vi "Average_Corner.vi"(7 "Average\nProjection":bool, 8 "Image":dbl[][](graph), 9 "Cursor C Coordinate":cluster{"X":dbl, "Y":dbl}, 10 "Cursor B Coordinate":cluster{"X":dbl, "Y":dbl}, 11 "Cursor A Coordinate":cluster{"X":dbl, "Y":dbl}) -> (0 "Cut image":dbl[][](graph), 1 "X-Axis":dbl[](array[numeric]), 2 "Intensity Average":dbl[](array[numeric]), 3 "Average\ncut image":dbl)   [LabVIEW 2014]
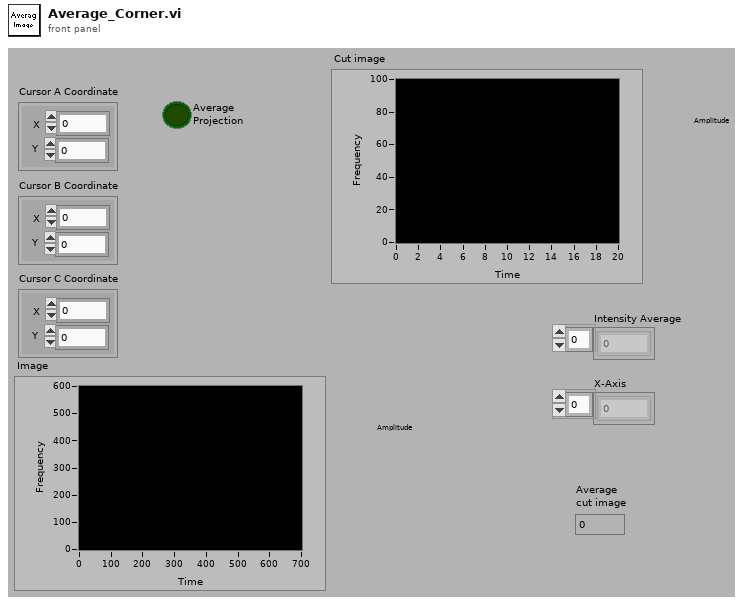
[diagram p1: front panel]
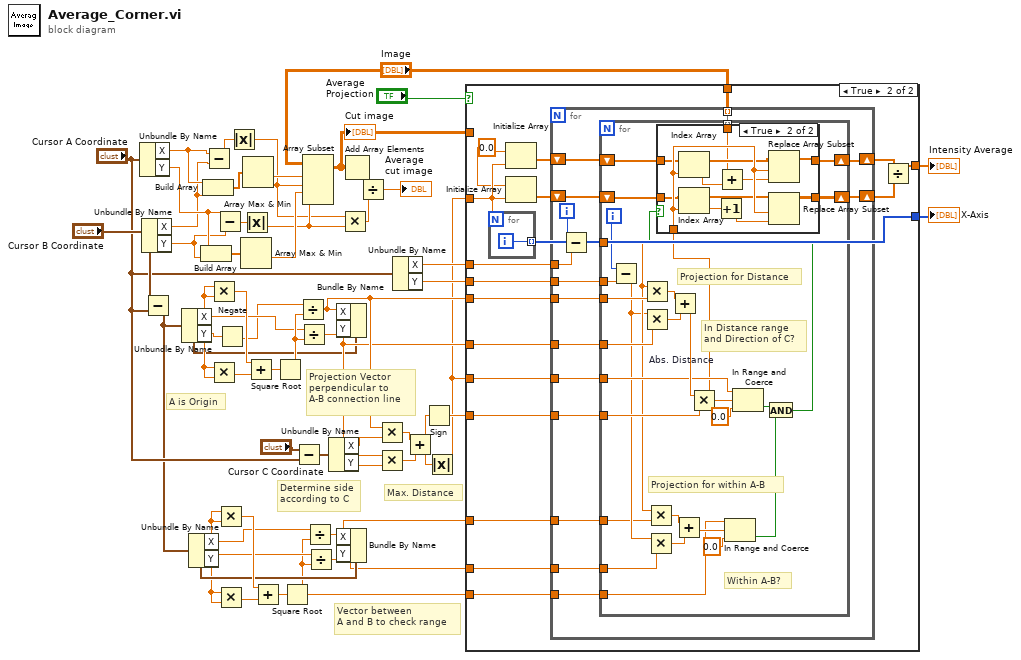
[diagram p0: block diagram]
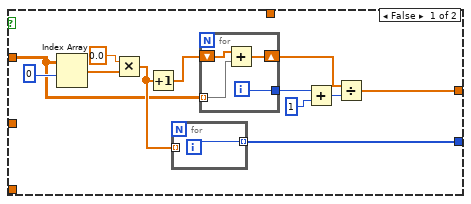
[diagram p2: hidden frame]
diagram:
  # "Vector between\nA and B to check range"
  # "Max. Distance"
  # "Determine side\naccording to C"
  # "A is Origin"
  # "Projection Vector\nperpendicular to \nA-B connection line"
  n1 = Unbundle By Name("Cursor A Coordinate") -> ("X"=w41:dbl, "Y"=w40:dbl)
  n2 = Unbundle By Name("Cursor B Coordinate") -> ("X"=w38:dbl, "Y"=w39:dbl)
  n3 = Subtract(x="Cursor B Coordinate", y="Cursor A Coordinate") -> (x-y=w10:cluster{"X":dbl, "Y":dbl})
  n4 = Unbundle By Name(w10) -> ("X"=w9:dbl, "Y"=w31:dbl)
  n5 = Unbundle By Name(w10) -> ("X"=w6:dbl, "Y"=w7:dbl)
  n6 = Build Array(w40, w39) -> (w50:dbl[])
  n7 = Build Array(w41, w38) -> (w51:dbl[])
  n8 = Subtract(x=w41, y=w38) -> (x-y=w46:dbl)
  n9 = Multiply(x=w9, y=w9) -> (x*y=w29:dbl)
  n10 = Multiply(x=w31, y=w31) -> (x*y=w30:dbl)
  n11 = Subtract(x=w40, y=w39) -> (x-y=w47:dbl)
  n12 = Multiply(x=w6, y=w6) -> (x*y=w11:dbl)
  n13 = Multiply(x=w7, y=w7) -> (x*y=w5:dbl)
  n14 = Negate(x=w31) -> (-x=w8:dbl)
  n15 = Absolute Value(x=w46) -> (abs(x)=w43:dbl)
  n16 = Array Max & Min(array=w50) -> (min value=w48:dbl)  [unwired: 3 out]
  n17 = Absolute Value(x=w47) -> (abs(x)=w44:dbl)
  n18 = Array Max & Min(array=w51) -> (min value=w49:dbl)  [unwired: 3 out]
  n19 = Add(x=w29, y=w30) -> (x+y=w28:dbl)
  n20 = Add(x=w11, y=w5) -> (x+y=w4:dbl)
  n21 = Square Root(x=w28) -> (sqrt(x)=w27:dbl)
  n22 = Square Root(x=w4) -> (sqrt(x)=w1:dbl)
  n23 = Subtract(x="Cursor C Coordinate", y="Cursor A Coordinate") -> (x-y=w20:cluster{"X":dbl, "Y":dbl})
  n24 = Divide(x=w8, y=w27) -> (x/y=w17:dbl)
  n25 = Divide(x=w9, y=w27) -> (x/y=w16:dbl)
  n26 = Array Subset(array="Image", index (row)=w49, length (row)=w43, index (col)=w48, length (col)=w44) -> (w36:dbl[][])
  "Cut image" <- w36
  n27 = Divide(x=w6, y=w1) -> (x/y=w3:dbl)
  n28 = Divide(x=w7, y=w1) -> (x/y=w2:dbl)
  n29 = Unbundle By Name(w20) -> ("X"=w18:dbl, "Y"=w19:dbl)
  n30 = Bundle By Name(cluster=w10, "X"=w17, "Y"=w16) -> ()  [unwired: 1 out]
  n31 = Bundle By Name(cluster=w10, "X"=w3, "Y"=w2) -> ()  [unwired: 1 out]
  n32 = Multiply(x=w43, y=w44) -> (x*y=w42:dbl)
  n33 = Add Array Elements(numeric array=w36) -> (sum=w45:dbl)
  n34 = Divide(x=w45, y=w42) -> (x/y=→"Average\ncut image":dbl)
  n35 = Multiply(x=w17, y=w18) -> (x*y=w22:dbl)
  n36 = Multiply(x=w16, y=w19) -> (x*y=w21:dbl)
  n37 = Unbundle By Name("Cursor A Coordinate") -> ("X"=w24:dbl, "Y"=w23:dbl)
  n38 = Add(x=w22, y=w21) -> (x+y=w14:dbl)
  n39 = Sign(1:w14) -> (0:w15:dbl)
  n40 = Absolute Value(x=w14) -> (abs(x)=w13:dbl)
  n41 = case shown="True" "Average\nProjection" {
    tunnel: w36 -> [w54 _]
    tunnel: [w53 w72] -> w35
    tunnel: [w52 w79] -> w34
    tunnel: w24 -> [_ w86]
    tunnel: w23 -> [_ w85]
    tunnel: w16 -> [_ w84]
    tunnel: w17 -> [_ w83]
    tunnel: w15 -> [_ w82]
    tunnel: w13 -> [_ w81]
    tunnel: w13 -> [_ w80]
    tunnel: "Image" -> [_ w75]
    tunnel: w3 -> [_ w71]
    tunnel: w2 -> [_ w70]
    tunnel: w1 -> [_ w69]
    frame False {
      n42 = Index Array(array=w54, index (row)=u32 0 ("Active Cursor")) -> (element=w56:dbl[])  [unwired: 1 in]
      n43 = Multiply(x=0.0 ("element"), y=w56) -> (x*y=w55:dbl[])
      n44 = Increment(x=w55) -> (x+1=w62:dbl[])
      n45 = for {
        tunnel: w55 -> [_] mode=indexing
        tunnel: [w64] -> w52 mode=indexing
        i -> [w64]
      }
      n46 = for {
        tunnel: w54 -> [w67] mode=indexing
        shift-right: [w66] -> w63
        shift-left: w62 -> [w68]
        tunnel: [w65] -> w59
        i -> [w65]
        n47 = Add(x=w68, y=w67) -> (x+y=w66:dbl[])
      }
      n48 = Add(x=w59, y=u32 1 ("Active Cursor")) -> (x+y=w61:u32)
      n49 = Divide(x=w63, y=w61) -> (x/y=w53:dbl[])
    }
    frame True {
      w76 = 0.0
      n50 = for {
        N: w80 -> [_]
        tunnel: [w87] -> w79 mode=indexing
        i -> [w87]
      }
      n51 = Initialize Array(w76, w80) -> (w78:dbl[])
      n52 = Initialize Array(w76, w80) -> (w77:dbl[])
      n53 = for {
        tunnel: w86 -> [w102]
        tunnel: w85 -> [w101]
        tunnel: w84 -> [w100]
        tunnel: w83 -> [w99]
        tunnel: w82 -> [w97]
        tunnel: w81 -> [w96]
        shift-right: [w92] -> w73
        shift-left: w77 -> [w94]
        shift-right: [w93] -> w74
        shift-left: w78 -> [w95]
        tunnel: w75 -> [w91] mode=indexing
        tunnel: w71 -> [w90]
        tunnel: w70 -> [w89]
        tunnel: w69 -> [w88]
        i -> [w103]
        n54 = Subtract(x=w103, y=w102) -> (x-y=w98:dbl)
        n55 = for {
          tunnel: w101 -> [w131]
          tunnel: w100 -> [w129]
          tunnel: w99 -> [w128]
          tunnel: w98 -> [w113]
          tunnel: w97 -> [w125]
          tunnel: w96 -> [w123]
          shift-right: [w121] -> w92
          shift-left: w94 -> [w120]
          shift-right: [w119] -> w93
          shift-left: w95 -> [w118]
          tunnel: w91 -> [w116] mode=indexing
          tunnel: w90 -> [w111]
          tunnel: w89 -> [w110]
          tunnel: w88 -> [w107]
          i -> [w130]
          # "Within A-B?"
          # "Projection for within A-B"
          # "In Distance range\nand Direction of C?"
          # "Projection for Distance"
          n56 = Subtract(x=w130, y=w131) -> (x-y=w112:dbl)
          n57 = Multiply(x=w113, y=w128) -> (x*y=w126:dbl)
          n58 = Multiply(x=w112, y=w129) -> (x*y=w127:dbl)
          n59 = Multiply(x=w113, y=w111) -> (x*y=w115:dbl)
          n60 = Multiply(x=w112, y=w110) -> (x*y=w114:dbl)
          n61 = Add(x=w126, y=w127) -> (x+y=w124:dbl)
          n62 = Add(x=w115, y=w114) -> (x+y=w108:dbl)
          n63 = Multiply "Abs. Distance"(x=w124, y=w125) -> (x*y=w117:dbl)
          n64 = In Range and Coerce(upper limit=w107, x=w108, lower limit=0.0) -> (In Range?=w105:bool)  [unwired: 1 out]
          n65 = In Range and Coerce(upper limit=w123, x=w117, lower limit=0.0) -> (In Range?=w106:bool)  [unwired: 1 out]
          n66 = And(x=w106, y=w105) -> (x .and. y?=w104:bool)
          n67 = case shown="True" w104 {
            tunnel: [w133 w134] -> w121
            tunnel: w120 -> [w133 w138]
            tunnel: [w132 w135] -> w119
            tunnel: w118 -> [w132 w137]
            tunnel: w117 -> [_ w143]
            tunnel: w116 -> [_ w136]
            frame False {
            }
            frame True {
              n68 = Index Array(array=w137, index=w143) -> (element=w141:dbl)
              n69 = Index Array(array=w138, index=w143) -> (element=w140:dbl)
              n70 = Increment(x=w140) -> (x+1=w139:dbl)
              n71 = Add(x=w136, y=w141) -> (x+y=w142:dbl)
              n72 = Replace Array Subset(array=w137, new element=w142, index=w143) -> (w135:dbl[])
              n73 = Replace Array Subset(array=w138, new element=w139, index=w143) -> (w134:dbl[])
            }
          }
        }
      }
      n74 = Divide(x=w74, y=w73) -> (x/y=w72:dbl[])
    }
  }
  "Intensity Average" <- w35
  "X-Axis" <- w34
